vi "Software PWM Output.vi"(5 "Duty Cycle":dbl=0.5 format="%.6f", 7 "Frequency":dbl=1.0 format="%.6f", 8 "error in":errorcluster, 9 "Output Terminal":tag="/Dev1/PFI12", 10 "Counter":tag="Dev1/ctr0", 11 "Refnum in":refnum<k21>) -> (0 "error out":errorcluster, 3 "Refnum out":refnum<k21>, 4 "Actual Duty Cycle":dbl, 6 "Actual Frequency":dbl)   [LabVIEW 2021]
uses:
  <vilib>/DAQmx/create/channels.llb/DAQmx Create Channel (CO-Pulse Generation-Frequency).vi
  <vilib>/DAQmx/configure/timing.llb/DAQmx Timing (Implicit).vi
  <resource>/objmgr/daqmx.rc
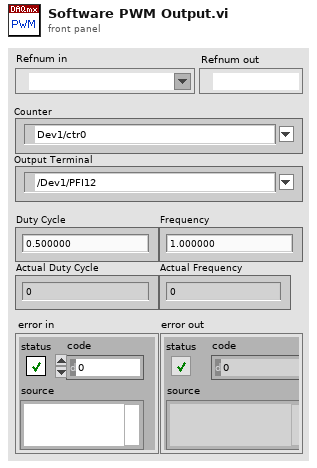
[diagram p1: front panel]
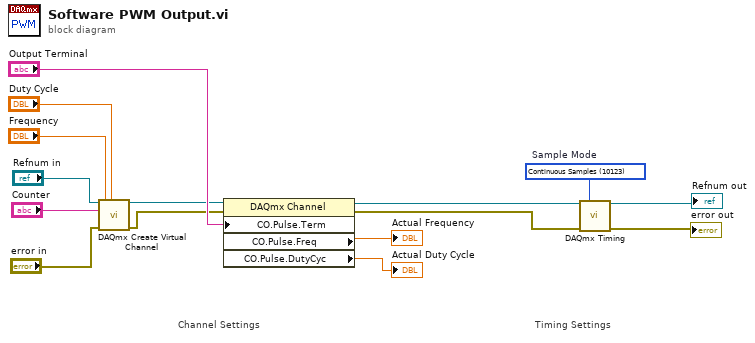
[diagram p0: block diagram]
diagram:
  w4 = 10123 items=["Finite Samples"=10178, "Continuous Samples"=10123, "Hardware Timed Single Point"=12522]  # Sample Mode
  # "Timing Settings"
  # "Channel Settings"
  n1 = call-poly <vilib>:"DAQmx Create Virtual Channel.vi"("task in"="Refnum in", "frequency"="Frequency", "duty cycle"="Duty Cycle", "counter"="Counter", "error in"="error in") -> ("task out"=w6:refnum<k21>, "error out"=w7:errorcluster)  [unwired: 9 in]
  n2 = property class="DAQmx Channel"(reference=w6, error in=w7, "CO.Pulse.Term"="Output Terminal") -> (reference out=w10:refnum<k21>, error out=w9:errorcluster, "CO.Pulse.Freq"=→"Actual Frequency":dbl, "CO.Pulse.DutyCyc"=→"Actual Duty Cycle":dbl)
  n3 = call-poly <vilib>:"DAQmx Timing.vi"("task/channels in"=w10, "sample mode"=w4, "error in"=w9) -> ("task out"=→"Refnum out":refnum<k21>, "error out"=→"error out":errorcluster)  [unwired: 11 in]
